vi "HaltTactic.vi"(6 "States in":enum16{"Halt", "Exit"}(ring), 8 "error in (no error)":errorcluster, 9 "Game in":refnum<class "Game.lvclass">, 10 "Robot":refnum<class "Robot.lvclass">, 11 "HaltTactic in":refnum<class "HaltTactic.lvclass">) -> (0 "error out":errorcluster, 2 "Robot out":refnum<class "Robot.lvclass">, 3 "HaltTactic out":refnum<class "HaltTactic.lvclass">)   [LabVIEW 2018, in "HaltTactic.lvclass"]
uses:
  HaltTactic.lvclass
  C:/Users/lucas/Documents/RoboIME/SSL_AI - pass/Tactic_class/Tactic.lvclass
  Robot_class/Robot.lvclass
  Game_class/Game.lvclass
  Tactic_class/Tactic.lvclass/Tactic.ctl
  Skillbook_class/Skillbook.lvclass/Skillbook.ctl
  HaltTactic.lvclass/HaltTactic.ctl
  Skillbook_class/Read HaltSkill.vi
  Tactic_class/Read Skillbook.vi
  Write States.vi
  Skillbook_class/Skillbook.lvclass
  HaltSkill_class/HaltSkill.lvclass
panel:
  out "x .or. y?":bool
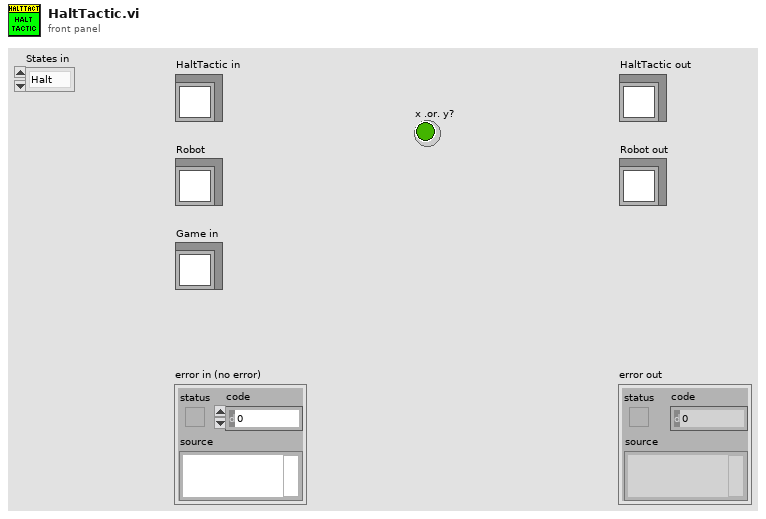
[diagram p1: front panel]
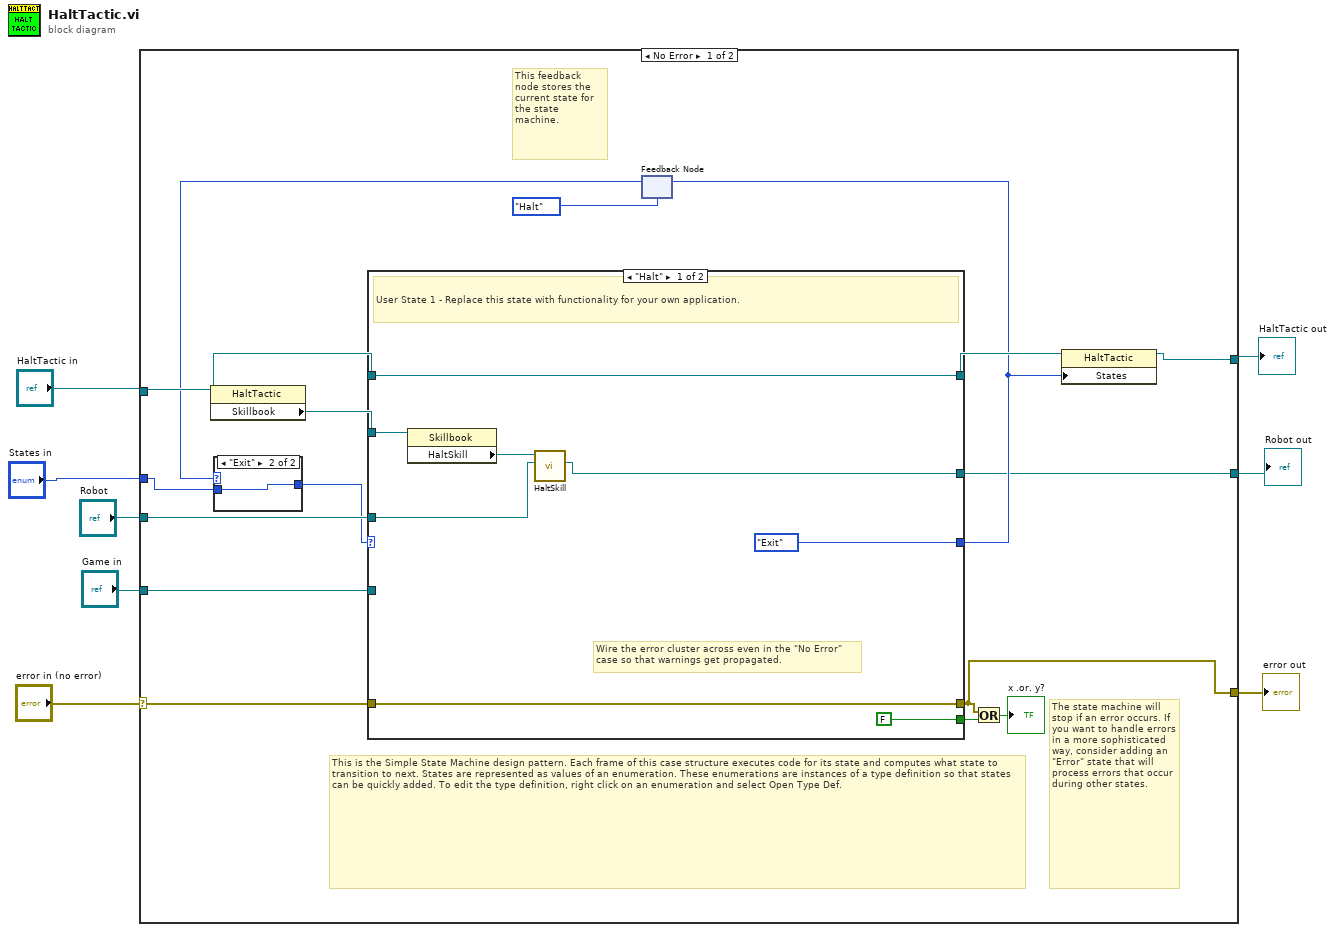
[diagram p0: block diagram]
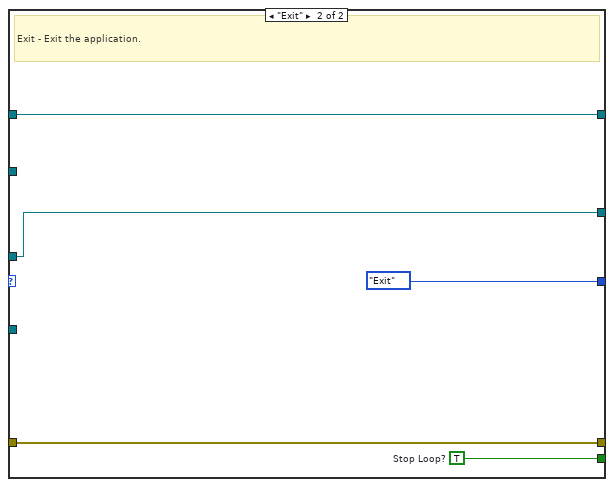
[diagram p3: hidden frame]
diagram:
  n1 = case shown="No Error" "error in (no error)" {
    selector: "error in (no error)" -> [w17 w42]
    tunnel: [w16 w42] -> w7
    tunnel: [w13 w41] -> w5
    tunnel: "HaltTactic in" -> [w20 w41]
    tunnel: "Robot" -> [w19 w40]
    tunnel: "Game in" -> [w18 _]
    tunnel: [w12 w40] -> w2
    tunnel: "States in" -> [w9 _]
    frame No Error {
      # "The state machine will stop if an error occurs. If you want to handle errors in a more sophisticated way, consider adding an \"Error\" state that will process errors that occur during other states."
      # "This feedback node stores the current state for the state machine."
      # "This is the Simple State Machine design pattern. Each frame of this case structure executes code for its state and computes what state to transition to next. States are represented as values of an enumeration. These enumerations are instances of a type definition so that states can be quickly added. To edit the type definition, right click on an enumeration and select Open Type Def."
      # "Wire the error cluster across even in the \"No Error\"\ncase so that warnings get propagated."
      n2 = property class="HaltTactic"(reference=w20) -> ("Skillbook"=w22:refnum<class "Skillbook.lvclass">)  [unwired: 1 in, 2 out]
      n3 = feedback #1(enum16{"Halt", "Exit"}."Halt" ("States")) -> (w11:enum16{"Halt", "Exit"})
      n4 = case shown="\"Exit\"" w11 {
        selector: w11 -> [w25 _]
        tunnel: [w25 w26] -> w10
        tunnel: w9 -> [_ w26]
        frame "Halt" {
        }
        frame "Exit" {
        }
      }
      n5 = case shown="\"Halt\"" w10 {
        tunnel: [enum16{"Halt", "Exit"}."Exit" ("States") enum16{"Halt", "Exit"}."Exit" ("States")] -> w14
        tunnel: [FALSE ("Stop Loop?") w39] -> w24
        tunnel: w22 -> [w33 _]
        tunnel: w19 -> [w30 w38]
        tunnel: [w29 w38] -> w12
        tunnel: [w32 w37] -> w21
        tunnel: w20 -> [w32 w37]
        tunnel: w18 -> [_ _]
        tunnel: [w28 w35] -> w16
        tunnel: w17 -> [w28 w35]
        frame "Halt" {
          # "User State 1 - Replace this state with functionality for your own application."
          n6 = property class="Skillbook"(reference=w33) -> ("HaltSkill"=w31:refnum<class "HaltSkill.lvclass">)  [unwired: 1 in, 2 out]
          n7 = call-dynamic "HaltSkill.vi"("Robot"=w30, "HaltSkill in"=w31) -> ("Robot out"=w29:refnum<class "Robot.lvclass">)  [unwired: 7 in, 2 out]
        }
        frame "Exit" {
          w39 = TRUE  # Stop Loop?
          # "Exit - Exit the application."
        }
      }
      n8 = feedback-in #1(w14) -> ()
      n9 = Or(x=w16, y=w24) -> (x .or. y?=→"x .or. y?":bool)
      n10 = property class="HaltTactic"(reference=w21, "States"=w14) -> (reference out=w13:refnum<class "HaltTactic.lvclass">)  [unwired: 1 in, 1 out]
    }
    frame Error {
    }
  }
  "error out" <- w7
  "HaltTactic out" <- w5
  "Robot out" <- w2
